vi "PacketGen_v2.vi"(0 "Hex Array":string[](array[string]), 1 "timings_offsets":dbl[](array[numeric]), 2 "distortion_corr":dbl, 5 "AOL_Globals":T2={"Imaging Protocol"=enum."AOL Z-Stack", "Number of POI"=0, "Number of Miniscans"=0, "Number of Trials"=0, "Number of Cycles "=0, "# Averaged Frames"=0, "Laser power (%)"=0, "Pockels (V)"=0.0, "Acquisition Length (sec)"=0.0, "Fill time (us)"=0.0, "POI Dwell time (us)"=0.0, "Miniscan Dwell time per pixel (us)"=0.0, "PMT 1"=0.0, "PMT 2"=0.0, "Back Apperture (mA)"=0.0, "Frame Size"=0, "Center Frequency"=0.0, "Field of View (um)"=175.0, "Field of View (norm)"=0.0, "DwellTime (us)"=0.0, "Ref Dwell Time (us)"=0.0, "Wavelength (nm)"=0.0, "Zoom"=0.0, "AOL Z"=0.0, "AOL Mode"=enum."Raster", "GridXY"=0.0, "GridZ"=0.0, "TriggerPeriod (sec)"=0.0, "Number of Pixels in Miniscan"=0, "Experiment folder path"=path "", "X centre"=0.0, "Y centre"=0.0, "Angle (degrees)"=0.0, "Angle Xs (degrees)"=0.0, "Angle Ys (degrees)"=0.0, "Plane Mode"=0, "Threshold"=[], "Regenerate Chirps"=FALSE, "Rectangle ROI length (pixels)"=0, "Rectangle ROI height (pixels)"=0, "AOD fill"=4900, "StartupDelay"=0, "Samples Wait after Trigger"=5080, "Slip Cycle"=600000, "Add Cycle"=TRUE, "Functional Mode"=enum."Point", "Z Start"=0.0, "Z Stop"=0.0, "# Planes"=0, "Total Pixels"=0, "Variable Miniscan Pixels"=[], "Use Variable Length"=FALSE, "Use Variable Resolution"=FALSE, "Laser power (%) at Z Start"=0, "Laser power (%) at Z Stop"=0, "Ref Z Step"=0} {"Angle Ys (degrees)" format="%#.6g"; "Angle Xs (degrees)" format="%#.6g"; "Plane Mode" items=["XY Plane", "XZ Plane", "YZ Plane", "arbitraryplane"]; "Frame Size" items=["100X100"=100, "128X128"=128, "200X200"=200, "256X256"=256, "512X512"=512, "1024x1024"=1024, "2048x2048"=2048]; "Back Apperture (mA)" format="%#.6g"; "Pockels (V)" format="%#.6g"; "PMT 2" format="%#.6g"; "PMT 1" format="%#.6g"; "Angle (degrees)" format="%#.6g"; "POI Dwell time (us)" format="%#.6g"}, 9 "Ny":i32, 11 "Nx":i32, 12 "Movement Correction":bool, 14 "Imaging Protocol":T1) -> (4 "HexPackets":string[](array[string]), 10 "Interrupted":bool, 13 "Repeat":i32, 15 "error out":errorcluster)   [LabVIEW 2020]
uses:
  Typedefs/Controls/AOL_Globals.ctl
  Typedefs/Imaging Protocols enum.ctl
  Typedefs/Frame Size.ctl
  Typedefs/AOL modes.ctl
  Typedefs/Plane Mode.ctl
  Typedefs/Functional Mode.ctl
  Global Variables/General Globals.vi
panel:
  out "Objective":i8=20
  in  "Protocol to save packets on":T1=enum."Functional Acquisition"
  in  "error in (no error)":errorcluster
  in  "Save Packets":bool
  out "Total Packets":i32
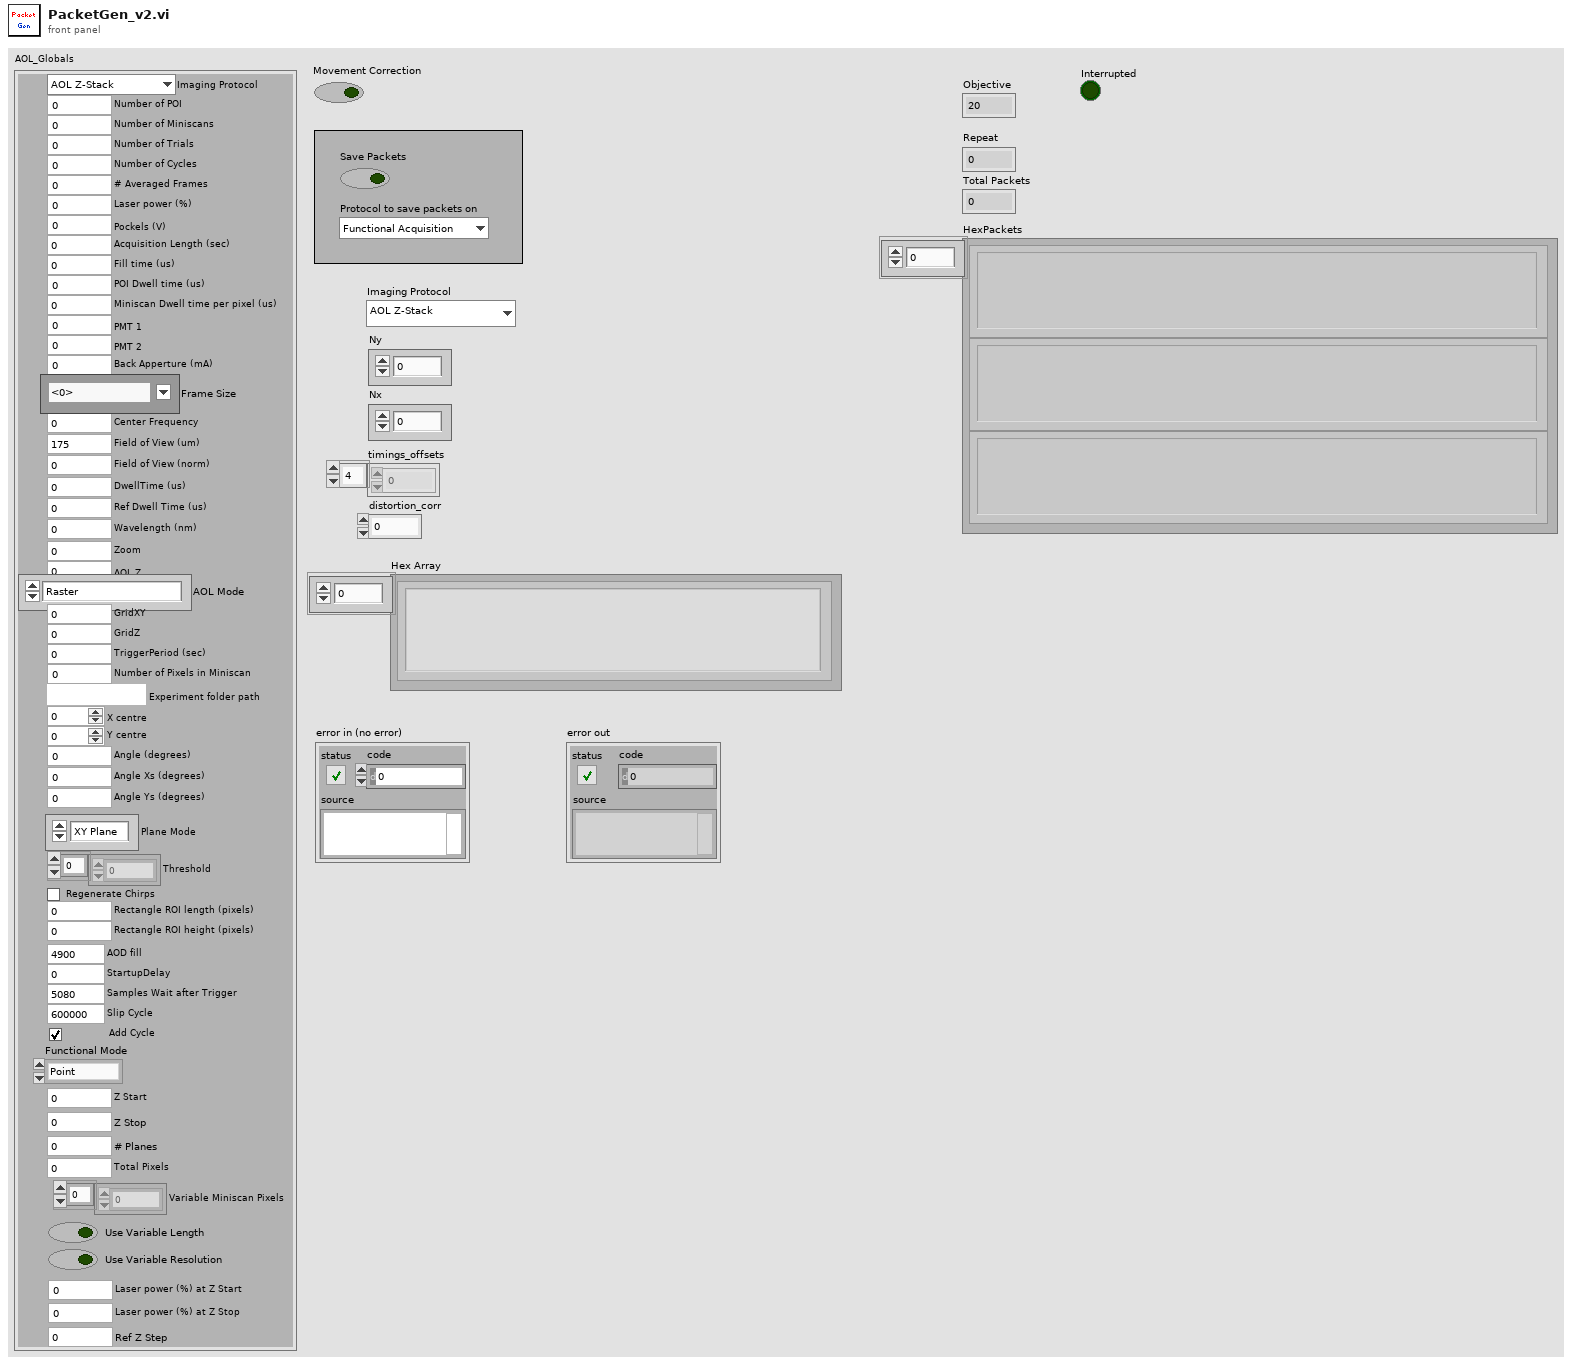
[diagram p1: front panel]
types:
  T1 = typedef "Imaging Protocols enum.ctl" = enum16{"AOL Z-Stack", "Motor Z Stack", "Parameter Sweep", "Functional Acquisition", "Single Plane Acquisition", "Volume Acquisition", "Live Imaging", "Live Plane Imaging", "Live Volume Imaging"}
  T2 = typedef "AOL_Globals.ctl" = cluster{"Imaging Protocol":T1, "Number of POI":u16, "Number of Miniscans":u16, "Number of Trials":u16, "Number of Cycles ":u64, "# Averaged Frames":u16, "Laser power (%)":u8, "Pockels (V)":dbl, "Acquisition Length (sec)":dbl, "Fill time (us)":dbl, "POI Dwell time (us)":dbl, "Miniscan Dwell time per pixel (us)":dbl, "PMT 1":dbl, "PMT 2":dbl, "Back Apperture (mA)":dbl, "Frame Size":T3, "Center Frequency":dbl, "Field of View (um)":dbl, "Field of View (norm)":dbl, "DwellTime (us)":dbl, "Ref Dwell Time (us)":dbl, "Wavelength (nm)":dbl, "Zoom":dbl, "AOL Z":dbl, "AOL Mode":T4, "GridXY":dbl, "GridZ":dbl, "TriggerPeriod (sec)":dbl, "Number of Pixels in Miniscan":u16, "Experiment folder path":path, "X centre":dbl, "Y centre":dbl, "Angle (degrees)":dbl, "Angle Xs (degrees)":dbl, "Angle Ys (degrees)":dbl, "Plane Mode":T5, "Threshold":u16[], "Regenerate Chirps":bool, "Rectangle ROI length (pixels)":u16, "Rectangle ROI height (pixels)":u16, "AOD fill":u16, "StartupDelay":i32, "Samples Wait after Trigger":u16, "Slip Cycle":u32, "Add Cycle":bool, "Functional Mode":T6, "Z Start":dbl, "Z Stop":dbl, "# Planes":i32, "Total Pixels":i32, "Variable Miniscan Pixels":u16[], "Use Variable Length":bool, "Use Variable Resolution":bool, "Laser power (%) at Z Start":u8, "Laser power (%) at Z Stop":u8, "Ref Z Step":i8}
  T3 = typedef "Frame Size.ctl" = u16
  T4 = typedef "AOL modes.ctl" = enum16{"Raster", "Structural", "Pointing", "Mini Scan", "Alignment"}
  T5 = typedef "Plane Mode.ctl" = u16
  T6 = typedef "Functional Mode.ctl" = enum16{"Point", "Line", "Patch", "Plane", "Volume"}
  T7 = typedef "Reference_Globals.ctl" = cluster{"Refrence data path":path, "Reference Rectangle":i16[][], "AOL Z":dbl, "No of pixels in a miniscan ":i32[], "Threshold":i16[], "No of miniscans":i32[], "Full Frame Size":u16, "Reference Image":T8, "dwelltime":dbl, "Zoom":dbl, "Field of View":dbl, "Z Step":i8, "Z pixels":i32, "Z Lines":u8, "Z Ignore":u8, "Laser":u8}
  T8 = typedef "IMAQ Image.ctl" = refnum<image>
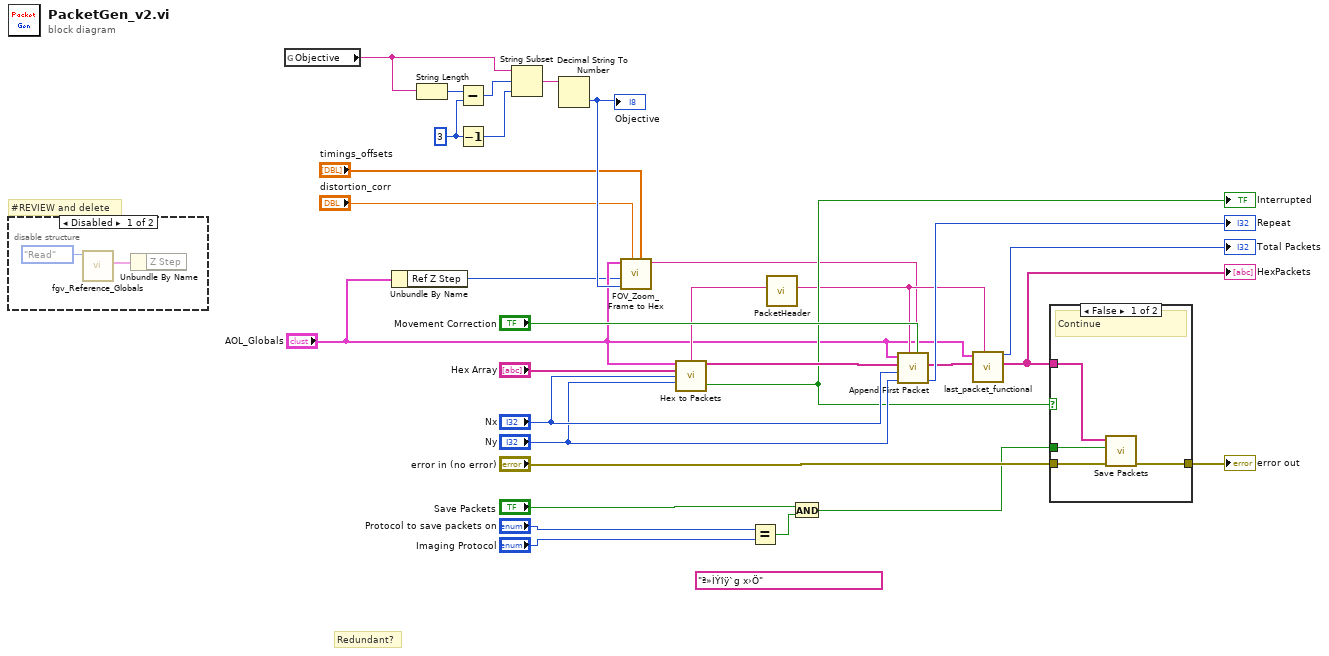
[diagram p0: block diagram]
diagram:
  w10 = 3
  (unwired) "ª»ÌÝîÿ`g x›Ö" ("PacketHeader")
  # "#REVIEW and delete"
  # "Redundant?"
  n1 = disable-structure shown="Disabled" {
    frame Disabled {
      n2 = call "fgv_Reference_Globals.vi"("Function"=enum16{"Intialize", "Write", "Read", "Clear"}."Read") -> ("Reference Data"=w31:T7)  [unwired: 9 in, 1 out]
      n3 = Unbundle By Name(w31) -> ()  [unwired: 1 out]
    }
    frame Enabled {
    }
  }
  n4 = global read "General Globals.vi" "Objective"() -> (w6:string)
  n5 = Unbundle By Name("AOL_Globals") -> ("Ref Z Step"=w1:i8)
  n6 = String Length(string=w6) -> (length=w9:i32)
  n7 = Subtract(x=w9, y=w10) -> (x-y=w11:i32)
  n8 = Decrement(x=w10) -> (x-1=w12:i32)
  n9 = String Subset(string=w6, offset (0)=w11, length (rest)=w12) -> (substring=w8:string)
  n10 = Decimal String To Number(string=w8) -> (number=w5:i32)  [unwired: 2 in, 1 out]
  "Objective" <- w5
  n11 = call "FOV_Zoom_Frame to Hex.vi"("timings_offsets"="timings_offsets", "distortion_corr"="distortion_corr", "Objective"=w5, "Z pixel Size"=w1, "AOL_Globals"="AOL_Globals") -> ("FOV-Zoom-FrameSize Hex"=w7:string)  [unwired: 6 in]
  n12 = Equal?(x="Protocol to save packets on", y="Imaging Protocol") -> (x = y?=w16:bool)
  n13 = call "PacketHeader.vi"() -> ("PacketHeader"=w13:string)  [unwired: 11 in]
  n14 = call "Hex to Packets.vi"("AOL_Globals"="AOL_Globals", "MAC Address"=w13, "Hex Array"="Hex Array", "Nx"="Nx", "Ny"="Ny") -> ("Packets"=w28:string[], "Interrupted"=w19:bool)  [unwired: 9 in]
  "Interrupted" <- w19
  n15 = And(x="Save Packets", y=w16) -> (x .and. y?=w14:bool)
  n16 = call "Append First Packet.vi"("Movement Correction"="Movement Correction", "FOV-Zoom-FrameSize Hex"=w7, "MAC Address"=w13, "Ny"="Ny", "Nx"="Nx", "Packets"=w28, "AOL_Globals"="AOL_Globals") -> ("Repeat"=→"Repeat":i32, "HexPackets"=w25:string[])  [unwired: 2 in, 1 out]
  n17 = call "last_packet_functional.vi"("MAC Address"=w13, "Packets"=w25, "AOL_Globals"="AOL_Globals") -> ("HexPackets"=w24:string[], "Total Packets"=→"Total Packets":i32)  [unwired: 6 in, 1 out]
  "HexPackets" <- w24
  n18 = case shown="False" w19 {
    tunnel: w14 -> [w36 _]
    tunnel: "error in (no error)" -> [w35 w37]
    tunnel: [w34 w37] -> w26
    tunnel: w24 -> [w33 _]
    frame False {
      # "Continue"
      n19 = call "Save Packets.vi"("error in (no error)"=w35, "Save Packets"=w36, "Packets in"=w33) -> ("error out"=w34:errorcluster)  [unwired: 8 in]
    }
    frame True {
      # "Interrupted"
    }
  }
  "error out" <- w26
